vi "Calculator.vi"(6 "Operation":T1, 9 "Y":dbl, 10 "X":dbl) -> (2 "Result":dbl)   [LabVIEW 2018]
uses:
  Operation--enum.ctl
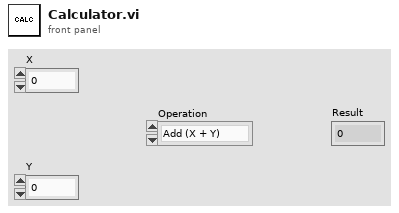
[diagram p1: front panel]
types:
  T1 = typedef "Operation--enum.ctl" = enum16{"Add (X + Y)", "Subtract (X - Y)", "Multiply (X * Y)", "Divide (X / Y)"}
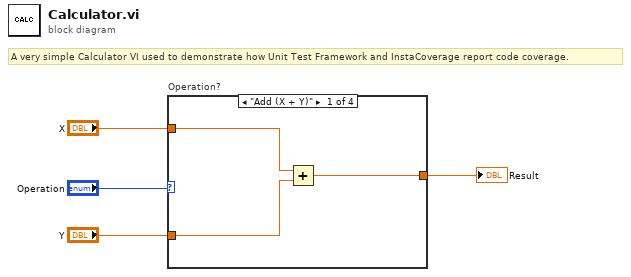
[diagram p0: block diagram]
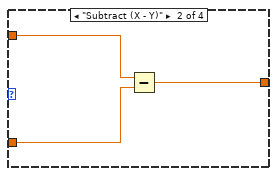
[diagram p2: hidden frame]
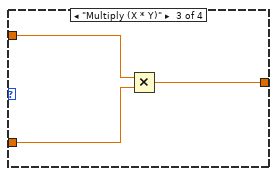
[diagram p3: hidden frame]
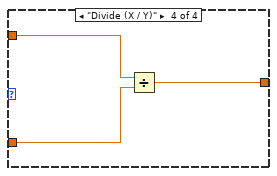
[diagram p4: hidden frame]
diagram:
  # "A very simple Calculator VI used to demonstrate how Unit Test Framework and InstaCoverage report code coverage."
  n1 = case "Operation?" shown="\"Add (X + Y)\"" "Operation" {
    tunnel: "X" -> [w7 w10 w13 w16]
    tunnel: "Y" -> [w6 w9 w12 w15]
    tunnel: [w5 w8 w11 w14] -> w1
    frame "Add (X + Y)" {
      n2 = Add(x=w7, y=w6) -> (x+y=w5:dbl)
    }
    frame "Subtract (X - Y)" {
      n3 = Subtract(x=w10, y=w9) -> (x-y=w8:dbl)
    }
    frame "Multiply (X * Y)" {
      n4 = Multiply(x=w13, y=w12) -> (x*y=w11:dbl)
    }
    frame "Divide (X / Y)" {
      n5 = Divide(x=w16, y=w15) -> (x/y=w14:dbl)
    }
  }
  "Result" <- w1
